vi "Begin.vi"(8 "error in":errorcluster) -> (0 "error out":errorcluster)   [LabVIEW 2014]
doc: "Called before other user functions, this VI is expected to open initial I/O refnums, load in file data, and do all program initialization. Notice that the <B>error out</B> terminal is simply used for data flow. Wiring it to other structures or subVIs ensures that this VI runs first."
uses:
  <vilib>/Rock Robotics/WPI/SafetyOutput/WPI_SafetyOutputConfigMenu.ctl
  <vilib>/Rock Robotics/WPI/DriverStation/WPI_DriverStationRobotMode2.ctl
  <vilib>/Rock Robotics/WPI/Joystick/WPI_JoystickDeviceEnum.ctl
  <vilib>/Rock Robotics/WPI/CAN/TalonSRX/WPI_CANTalonSRX_APIControlMode.ctl
  <vilib>/Rock Robotics/SystemInterfaces/DIO/FPGA_DIOChannel.ctl
  <vilib>/Rock Robotics/WPI/CAN/TalonSRX/WPI_CANTalonSRX_APIFeedbackSelect.ctl
  Robot Global Data.vi
  <vilib>/Rock Robotics/Network Tables/SD Write String Array.vi
  <vilib>/Rock Robotics/WPI/RobotDrive/WPI_RobotDriveOpen4MotorWithCANTalonSRX.vi
  <vilib>/Rock Robotics/WPI/MotorControl/WPI_MotorControlOpenCANTalonSRX.vi
  <vilib>/Rock Robotics/WPI/RobotDrive/WPI_RobotDriveOpen2MotorWithCANTalonSRX.vi
  <vilib>/Rock Robotics/WPI/Counter/WPI_CounterDigitalInputToDigitalSource.vi
  <vilib>/Rock Robotics/WPI/Compressor/WPI_CompressorGetSetRefNum.vi
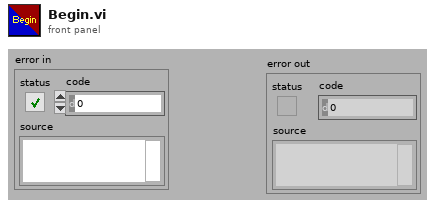
[diagram p1: front panel]
types:
  T1 = typedef "WPI_CANTalonSRX_APIFeedbackSelect.ctl" = enum16{"Digital Quadrature Encoder", "Analog Potentiometer", "Analog Encoder"}
  T2 = typedef "FPGA_DIOChannel.ctl" = enum8{"DIO 0", "DIO 1", "DIO 2", "DIO 3", "DIO 4", "DIO 5", "DIO 6", "DIO 7", "DIO 8", "DIO 9", "DIO MXP 0", "DIO MXP 1", "DIO MXP 2", "DIO MXP 3", "DIO MXP 4", "DIO MXP 5", "DIO MXP 6", "DIO MXP 7", "DIO MXP 8", "DIO MXP 9", "DIO MXP 10", "DIO MXP 11", "DIO MXP 12", "DIO MXP 13", "DIO MXP 14", "DIO MXP 15", "Invalid"}
  T3 = typedef "WPI_CANTalonSRX_APIControlMode.ctl" = enum8{"Percent VBus", "Speed", "Position", "Slave", "Unchanged / Invalid"}
  T4 = typedef "WPI_JoystickDeviceEnum.ctl" = enum16{"USB 0", "USB 1", "USB 2", "USB 3", "USB 4", "USB 5"}
  T5 = typedef "WPI_DriverStationRobotMode2.ctl" = enum16{"Autonomous Disabled", "Autonomous Enabled", "Teleop Disabled", "Teleop Enabled", "Disconnected", "Finish", "Test Disabled", "Test Enabled", "Emergency Stopped"}
  T6 = typedef "WPI_SafetyOutputConfigMenu.ctl" = enum16{"Enable", "Disable"}
  T7 = typedef "WPI_JoystickDevRef.ctl" = cluster{"Device":T4}
  T8 = typedef "WPI_DigitalInputDevRef.ctl" = cluster{"DevStatus":errorcluster, "DIO Channel":T2, "Controller":T9}
  T9 = typedef "FPGA_TypedefDigitalModule.ctl" = enum16{"Controller 1"}
  T10 = typedef "FPGA_CounterEncoderSourceConvertionLVSourceType.ctl" = cluster{"DevStatus":errorcluster, "AnalogTriggerMode?":bool, "DigitalMode":cluster{"Controller":T9, "DIO Channel":T11}, "AnalogTriggerMode":cluster{"AnalogTriggerIndex":T12, "OutputType":T13}}
  T11 = typedef "FPGA_DIODigitalSourceChannel.ctl" = enum8{"DIO 0", "DIO 1", "DIO 2", "DIO 3", "DIO 4", "DIO 5", "DIO 6", "DIO 7", "DIO 8", "DIO 9", "DIO MXP 0", "DIO MXP 1", "DIO MXP 2", "DIO MXP 3", "DIO MXP 4", "DIO MXP 5", "DIO MXP 6", "DIO MXP 7", "DIO MXP 8", "DIO MXP 9", "DIO MXP 10", "DIO MXP 11", "DIO MXP 12", "DIO MXP 13", "DIO MXP 14", "DIO MXP 15", "Disabled"}
  T12 = typedef "FPGA_AnalogTriggerIndex.ctl" = enum8{"Trig 0", "Trig 1", "Trig 2", "Trig 3", "Trig 4", "Trig 5", "Trig 6", "Trig 7", "Invalid"}
  T13 = typedef "FPGA_AnalogTriggerOutType.ctl" = enum16{"InWindow", "TriggerState", "Rising", "Falling"}
  T14 = typedef "WPI_RobotDriveDevRef.ctl" = cluster{"DevStatus":errorcluster, "Motors[]":T15[], "Square Inputs":bool, "Max Output":dbl}
  T15 = typedef "WPI_MotorControlDeviceRef.ctl" = cluster{"DeviceStatus":errorcluster, "Type":T16, "PWM":cluster{"Controller":T9, "PWM Channel":T17, "DeadBand":T18}, "CAN":cluster{"Device Number":u8, "Control Mode":T19, "Semaphore":T20, "Max Vout":dbl, "TalonSRX Control Mode":T3}, "Invert":bool, "TransformRef":T21, "InvTransformRef":T21}
  T16 = typedef "WPI_MotorControlType.ctl" = enum16{"PWM", "CAN", "CANTalonSRX"}
  T17 = typedef "FPGA_DIOPWMChannel.ctl" = enum8{"PWM 0", "PWM 1", "PWM 2", "PWM 3", "PWM 4", "PWM 5", "PWM 6", "PWM 7", "PWM 8", "PWM 9", "PWM MXP 0", "PWM MXP 1", "PWM MXP 2", "PWM MXP 3", "PWM MXP 4", "PWM MXP 5", "PWM MXP 6", "PWM MXP 7", "PWM MXP 8", "PWM MXP 9", "Invalid"}
  T18 = typedef "WPI_PWMDeadband.ctl" = cluster{"Name":string, "maxPositivePwm":i32, "minPositivePwm":i32, "centerPwm":i32, "maxNegativePwm":i32, "minNegativePwm":i32, "angularRange":u16}
  T19 = typedef "WPI_CANJaguar_ControlMode.ctl" = enum8{"Percent VBus", "Current", "Speed", "Position", "Voltage"}
  T20 = typedef "Semaphore RefNum" = refnum<k1>
  T21 = typedef "WPI_PWMTransform_ConPane.ctl" = refnum<vi>
  T22 = typedef "WPI_EncoderDevRef.ctl" = cluster{"DevStatus":errorcluster, "EncoderIndex":T23, "CounterIndex":T24, "DistancePerCount":dbl, "Decoding Type":T25}
  T23 = typedef "FPGA_EncoderIdx.ctl" = enum8{"Enc 0", "Enc 1", "Enc 2", "Enc 3", "Enc 4", "Enc 5", "Enc 6", "Enc 7", "Invalid"}
  T24 = typedef "FPGA_CounterCtrSystemIndex.ctl" = enum8{"Ctr 0", "Ctr 1", "Ctr 2", "Ctr 3", "Ctr 4", "Ctr 5", "Ctr 6", "Ctr 7", "Invalid"}
  T25 = typedef "WPI_EncoderType.ctl" = enum16{"1x", "2x", "4x"}
  T26 = typedef "WPI_CompressorDevRef.ctl" = cluster{"DevStatus":errorcluster, "Pneumatics Control Module":u8}
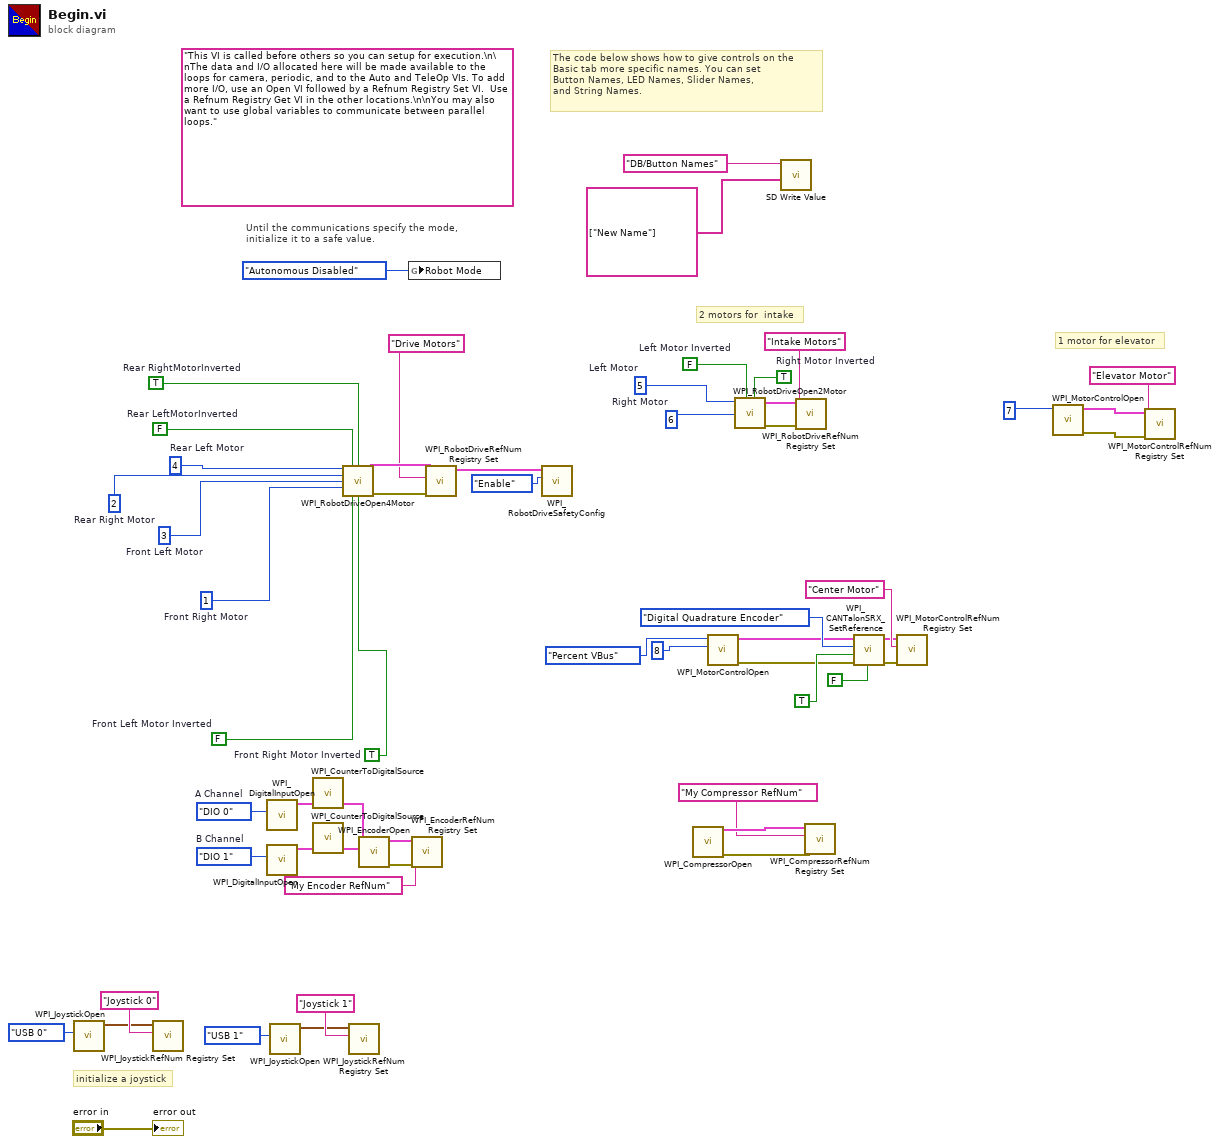
[diagram p0: block diagram]
diagram:
  w19 = FPGA_DIOChannel."DIO 1"  # B Channel
  w18 = FPGA_DIOChannel."DIO 0"  # A Channel
  w20 = TRUE  # Right Motor Inverted
  w21 = FALSE  # Left Motor Inverted
  w26 = u8 6  # Right Motor
  w27 = u8 5  # Left Motor
  w33 = u8 1  # Front Right Motor
  w34 = u8 3  # Front Left Motor
  w35 = u8 2  # Rear Right Motor
  w36 = u8 4  # Rear Left Motor
  w41 = TRUE  # Front Right Motor Inverted
  w42 = FALSE  # Front Left Motor Inverted
  (unwired) "This VI is called before others so you can setup for execution.\n\nThe data and I/O allocated here will be made available to the loops for camera, periodic, and to the Auto and TeleOp VIs. To add more I/O, use an Open VI followed by a Refnum Registry Set VI.  Use a Refnum Registry Get VI in the other locations.\n\nYou may also want to use global variables to communicate between parallel loops."
  w55 = FALSE  # Rear LeftMotorInverted
  w56 = TRUE  # Rear RightMotorInverted
  # "2 motors for  intake"
  # "1 motor for elevator"
  # "The code below shows how to give controls on the\nBasic tab more specific names. You can set\nButton Names, LED Names, Slider Names,\nand String Names."
  # "initialize a joystick"
  # "Until the communications specify the mode,\ninitialize it to a safe value."
  n1 = call <vilib>:"WPI_JoystickOpen.vi"("JoystickDevice"=WPI_JoystickDeviceEnum."USB 0") -> ("JoystickDevRef"=w47:T7)  [unwired: 10 in]
  n2 = call <vilib>:"WPI_JoystickRefNum Registry Set.vi"("refnum name"="Joystick 0", "JoystickDevRef"=w47) -> ()  [unwired: 8 in, 2 out]
  n3 = call <vilib>:"WPI_DigitalInputOpen.vi"("DIO Channel"=w18) -> ("DigitalInputDevRef"=w15:T8)  [unwired: 2 in, 8 out]
  n4 = call <vilib>:"WPI_DigitalInputOpen.vi"("DIO Channel"=w19) -> ("DigitalInputDevRef"=w16:T8)  [unwired: 2 in, 8 out]
  n5 = call <vilib>:"WPI_JoystickOpen.vi"("JoystickDevice"=WPI_JoystickDeviceEnum."USB 1") -> ("JoystickDevRef"=w38:T7)  [unwired: 10 in]
  n6 = call-poly <vilib>:"WPI_CounterToDigitalSource.vi"("DigitalInputDevRef"=w15) -> ("Digital Source"=w14:T10)  [unwired: 6 out]
  n7 = call-poly <vilib>:"WPI_CounterToDigitalSource.vi"("DigitalInputDevRef"=w16) -> ("Digital Source"=w17:T10)  [unwired: 6 out]
  n8 = call-poly <vilib>:"WPI_RobotDriveOpen4Motor.vi"("Rear Left Motor"=w36, "Rear Left Motor Inverted"=w55, "Rear Right Motor Inverted"=w56, "Rear Right Motor"=w35, "Front Left Motor"=w34, "Front Right Motor"=w33, "Front Left Motor Inverted"=w42, "Front Right Motor Inverted"=w41) -> ("RobotDriveDevRef"=w54:T14, "error out"=w52:errorcluster)  [unwired: 6 in]
  n9 = call <vilib>:"WPI_JoystickRefNum Registry Set.vi"("refnum name"="Joystick 1", "JoystickDevRef"=w38) -> ()  [unwired: 8 in, 2 out]
  n10 = call <vilib>:"WPI_EncoderOpen.vi"("BSource"=w17, "ASource"=w14) -> ("error out"=w13:errorcluster, "EncoderDevRef"=w12:T22)  [unwired: 6 in, 2 out]
  n11 = global write "Robot Global Data.vi" "Robot Mode"(WPI_DriverStationRobotMode2."Autonomous Disabled" ("Robot Mode")) -> ()
  n12 = call <vilib>:"WPI_EncoderRefNum Registry Set.vi"("error in (no error)"=w13, "refnum name"="My Encoder RefNum", "EncoderDevRef"=w12) -> ()  [unwired: 7 in, 2 out]
  n13 = call <vilib>:"WPI_RobotDriveRefNum Registry Set.vi"("error in (no error)"=w52, "refnum name"="Drive Motors", "RobotDriveDevRef"=w54) -> ("RobotDriveDevRef"=w51:T14)  [unwired: 8 out]
  n14 = call <vilib>:"WPI_RobotDriveSafetyConfig.vi"("mode"=WPI_SafetyOutputConfigMenu."Enable", "RobotDriveDevRef"=w51) -> ()  [unwired: 8 in, 2 out]
  n15 = call <vilib>:"WPI_CompressorOpen.vi"() -> ("CompressorDevRef"=w2:T26, "error out"=w3:errorcluster)  [unwired: 14 in]
  n16 = call-poly <vilib>:"WPI_MotorControlOpen.vi"("Device Number"=u8 8, "Control Mode"=WPI_CANTalonSRX_APIControlMode."Percent VBus") -> ("error out"=w4:errorcluster, "MotorControlDeviceRef"=w7:T15)  [unwired: 8 in]
  n17 = call-poly <vilib>:"WPI_RobotDriveOpen2Motor.vi"("Right Motor Inverted"=w20, "Left Motor Inverted"=w21, "Right Motor"=w26, "Left Motor"=w27) -> ("error out"=w29:errorcluster, "RobotDriveDevRef"=w30:T14)  [unwired: 6 in]
  n18 = call-poly <vilib>:"SD Write Value.vi"("String Array"=string[] ["New Name"], "Name"="DB/Button Names") -> ()  [unwired: 8 in, 2 out]
  n19 = call <vilib>:"WPI_RobotDriveRefNum Registry Set.vi"("error in (no error)"=w29, "refnum name"="Intake Motors", "RobotDriveDevRef"=w30) -> ()  [unwired: 7 in, 2 out]
  n20 = call <vilib>:"WPI_CompressorRefNum Registry Set.vi"("error in (no error)"=w3, "refnum name"="My Compressor RefNum", "CompressorDevRef"=w2) -> ()  [unwired: 7 in, 2 out]
  n21 = call <vilib>:"WPI_CANTalonSRX_SetReference.vi"("Reverse Closed-Loop Output"=FALSE, "error in (no error)"=w4, "Reverse Feedback Sensor"=TRUE, "Feedback Reference"=WPI_CANTalonSRX_APIFeedbackSelect."Digital Quadrature Encoder", "CAN Talon SRX Ref"=w7) -> ("error out"=w5:errorcluster, "CAN Talon SRX Ref Out"=w6:T15)  [unwired: 5 in]
  n22 = call <vilib>:"WPI_MotorControlRefNum Registry Set.vi"("error in (no error)"=w5, "refnum name"="Center Motor", "MotorControlDevRef"=w6) -> ()  [unwired: 7 in, 2 out]
  n23 = call-poly <vilib>:"WPI_MotorControlOpen.vi"("Device Number"=u8 7) -> ("error out"=w25:errorcluster, "MotorControlDeviceRef"=w24:T15)  [unwired: 9 in]
  n24 = call <vilib>:"WPI_MotorControlRefNum Registry Set.vi"("error in (no error)"=w25, "refnum name"="Elevator Motor", "MotorControlDevRef"=w24) -> ()  [unwired: 7 in, 2 out]
  "error out" <- "error in"
